vi "Readable Class Name.vi"(10 "Full class name":string="Generic Digital Multi Meter.lvlib:Tektronix DMM4020.lvlib:Tektronix DMM4020.lvclass") -> (2 "Proper Readable Class Name":string)   [LabVIEW 2016, in "SetUp VIs.lvlib"]
uses:
  SetUp VIs.lvlib
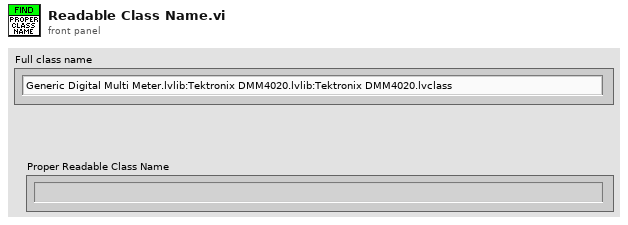
[diagram p1: front panel]
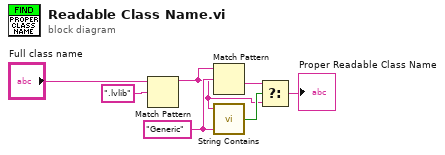
[diagram p0: block diagram]
diagram:
  w5 = "Generic" ("regular expression")
  n1 = Match Pattern(string="Full class name", regular expression=".lvlib") -> (before substring=w2:string)  [unwired: 1 in, 3 out]
  n2 = Match Pattern(string=w2, regular expression=w5) -> (after substring=w3:string)  [unwired: 1 in, 3 out]
  n3 = call "String Contains.vi"("Regular expression"=w5, "Input String"=w2) -> ("Found?"=w4:bool)  [unwired: 2 in, 1 out]
  n4 = Select(t=w3, s=w4, f=w2) -> (s? t:f=→"Proper Readable Class Name":string)
